vi "[Instrument] Close All.vi"() -> ()   [LabVIEW 2021]
panel:
  in  "Close All session":bool
  in  "Stop":bool
  out "instrument handle":refnum<k15>
  out "DropDownList[]":string[](array[string])
  # "VISA Sessions"
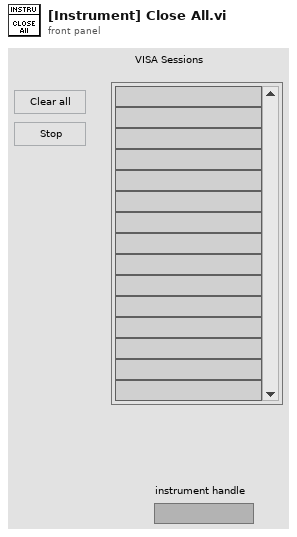
[diagram p1: front panel]
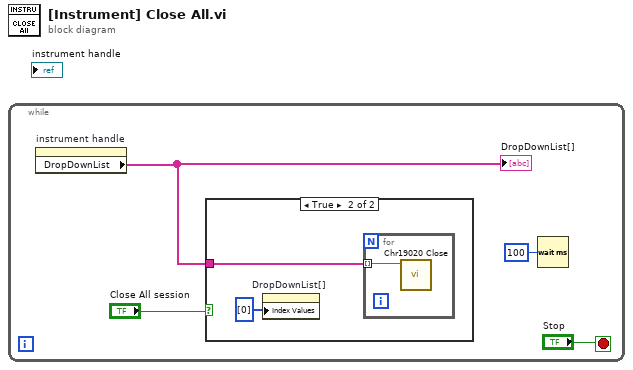
[diagram p0: block diagram]
diagram:
  n1 = while {
    stop <- "Stop" stop-if-true
    n2 = property on="instrument handle" class="IVIName"() -> ("DropDownList"=w2:string[])  [unwired: 2 in, 2 out]
    "DropDownList[]" <- w2
    n3 = case shown="True" "Close All session" {
      tunnel: w2 -> [_ w6]
      frame False {
      }
      frame True {
        n4 = property on="DropDownList[]" class="Arr (strict)"("Index Values"=u32[] [0]) -> ()  [unwired: 2 in, 2 out]
        n5 = for {
          tunnel: w6 -> [w7] mode=indexing
          n6 = call <instrlib>:"Chr19020 Close.vi"("instrument handle"=w7) -> ()  [unwired: 10 in, 1 out]
        }
      }
    }
    n7 = Wait (ms)(milliseconds to wait=u32 100) -> ()  [unwired: 1 out]
  }
